vi "TestGetArrayFromMatlab.vi"() -> ()   [LabVIEW 2017]
uses:
  Types/MatlabDataBundle.ctl
  Types/MatlabDataType.ctl
panel:
  out "Value":variant
  in  "Read":bool
  out "Matlab param data":T1[](array[typedef])
  out "Read String array":string[](array[string])
  in  "Temp ID":dbl
  out "erros?":bool
  out "ExpID":string="Exp77c27ca2690b43b31b68791e85e1b449C"
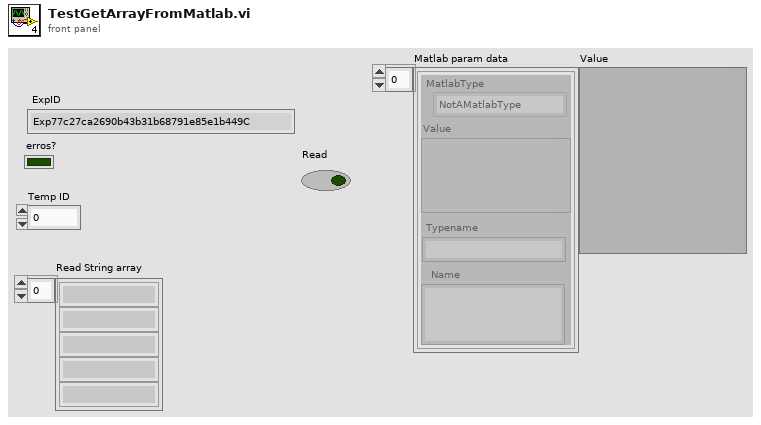
[diagram p1: front panel]
types:
  T1 = typedef "MatlabDataBundle.ctl" = cluster{"MatlabType":T2, "Value":variant, "Name":string, "Typename":string}
  T2 = typedef "MatlabDataType.ctl" = enum16{"NotAMatlabType", "Real", "Complex", "String", "Boolean"}
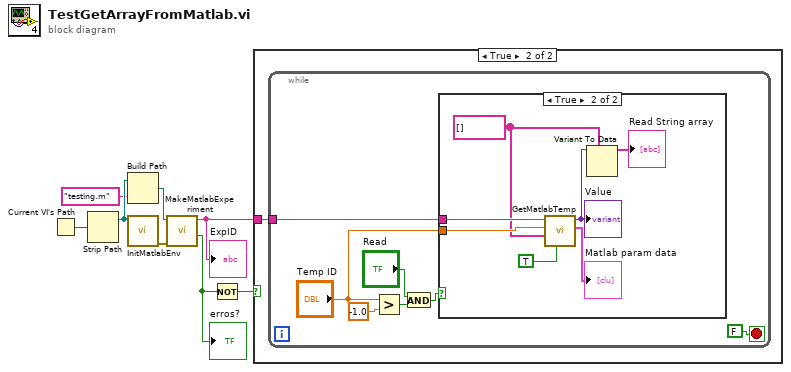
[diagram p0: block diagram]
diagram:
  n1 = Current VI's Path() -> (path=w5:path)
  n2 = Strip Path(path=w5) -> (stripped path=w7:path)  [unwired: 1 out]
  n3 = Build Path(base path=w7, name or relative path="testing.m") -> (appended path=w8:path)
  n4 = call "InitMatlabEnv.vi"("Working directory"=w7) -> ("error out"=w6:errorcluster)  [unwired: 10 in]
  n5 = call "MakeMatlabExperiment.vi"("error in"=w6, "experimentFilepath"=w8) -> ("erros?"=w3:bool, "ExpID"=w2:string)  [unwired: 6 in, 2 out]
  "ExpID" <- w2
  "erros?" <- w3
  n6 = Not(x=w3) -> (.not. x?=w1:bool)
  n7 = case shown="True" w1 {
    tunnel: w2 -> [_ w9]
    frame False {
    }
    frame True {
      n8 = while {
        tunnel: w9 -> [w13]
        stop <- FALSE stop-if-true
        n9 = Greater?(x="Temp ID", y=-1.0) -> (0:w15:bool)
        n10 = And(x="Read", y=w15) -> (x .and. y?=w14:bool)
        n11 = case shown="True" w14 {
          tunnel: w13 -> [_ w23]
          tunnel: "Temp ID" -> [_ w22]
          frame False {
          }
          frame True {
            w19 = string[] [] ("StringAr")
            n12 = call "GetMatlabTemp.vi"("IgnoreContainerName"=TRUE, "Value Tp Update (or type)"=w19, "index in"=w22, "ExpID"=w23) -> ("Matlab param data"=→"Matlab param data":T1[], "Value"=w21:variant)  [unwired: 5 in, 1 out]
            "Value" <- w21
            n13 = Variant To Data(type=w19, Variant=w21) -> (data=→"Read String array":string[])  [unwired: 1 in, 1 out]
          }
        }
      }
    }
  }
